vi "_Read.vi"(8 "error in (no error)":errorcluster, 11 "Lockin and Fluke Multimeter in":refnum<class "Lockin and Fluke Multimeter.lvclass">) -> (0 "error out":errorcluster, 2 "X array":T1, 3 "Lockin and Fluke Multimeter out":refnum<class "Lockin and Fluke Multimeter.lvclass">)   [LabVIEW 2017, in "Lockin and Fluke Multimeter.lvclass"]
doc: "(Protected, Dynamic, Pure Virtual/Abstract) Perform a measurement and return one or more channels of data. Outsiders should not call this method, but instead the public \"Read Data.vi\"."
uses:
  Lockin and Fluke Multimeter.lvclass
  Utility Classes/Readable/X array.ctl
  Utility Classes/Readable/X.ctl
  Lockin and Fluke Multimeter.lvclass/Lockin and Fluke Multimeter.ctl
  Lockin/sr830/SR830.lvlib
  Fluke Multimeter/Fluke 8840/Fluke 8840.lvlib
  Utility Classes/Readable/Readable.lvclass
panel:
  out "Ratio multiplier":dbl
  out "Fluke multiplier":dbl
  out "Lockin multiplier":dbl
  out "Fluke measurement":dbl format="%^.6e"
  out "R":dbl
  out "Y":dbl
  out "X":dbl
  out "trigger mode (0:internal)":u16(ring) items=["internal - continuous trigger", "external - rear panel trigger with delay", "external - bus trigger with delay", "external - rear panel trigger", "external - bus trigger"]
  out "rate (0:slow)":u16(ring) items=["slow", "medium", "fast"]
  out "range (0:auto)":u16(ring) items=["autorange", "200mV, 200 ohms", "2V, 2 kohms", "20V, 20 kohms", "200V, 200 kohms", "1000Vdc, 700 Vac, 2 Mohms", "20 Mohms"]
  out "function (0:volts DC)":u16(ring) items=["volts DC", "volts AC", "2-wire k.ohms", "4-wire k.ohms", "mA DC", "mA AC"]
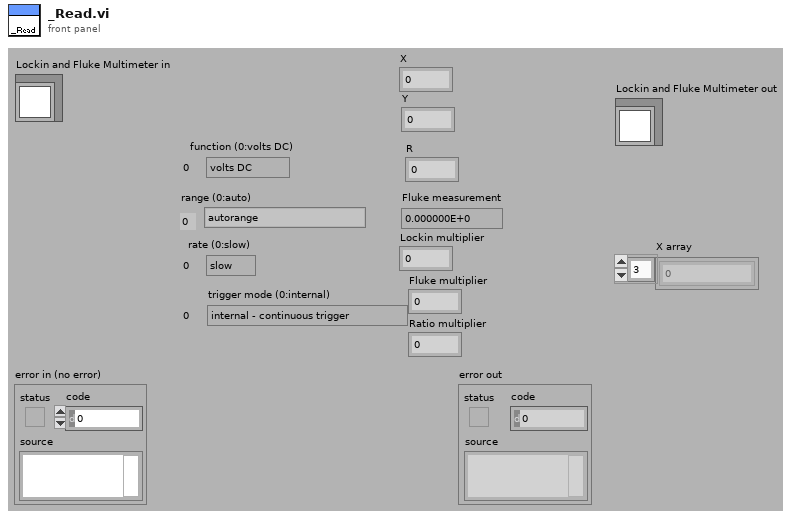
[diagram p1: front panel]
types:
  T1 = typedef "Readable.lvclass/X array.ctl" = T2[]
  T2 = typedef "Readable.lvclass/X.ctl" = dbl
  T3 = typedef "Lockin SR830.lvclass/Sensitivity.ctl" = u16
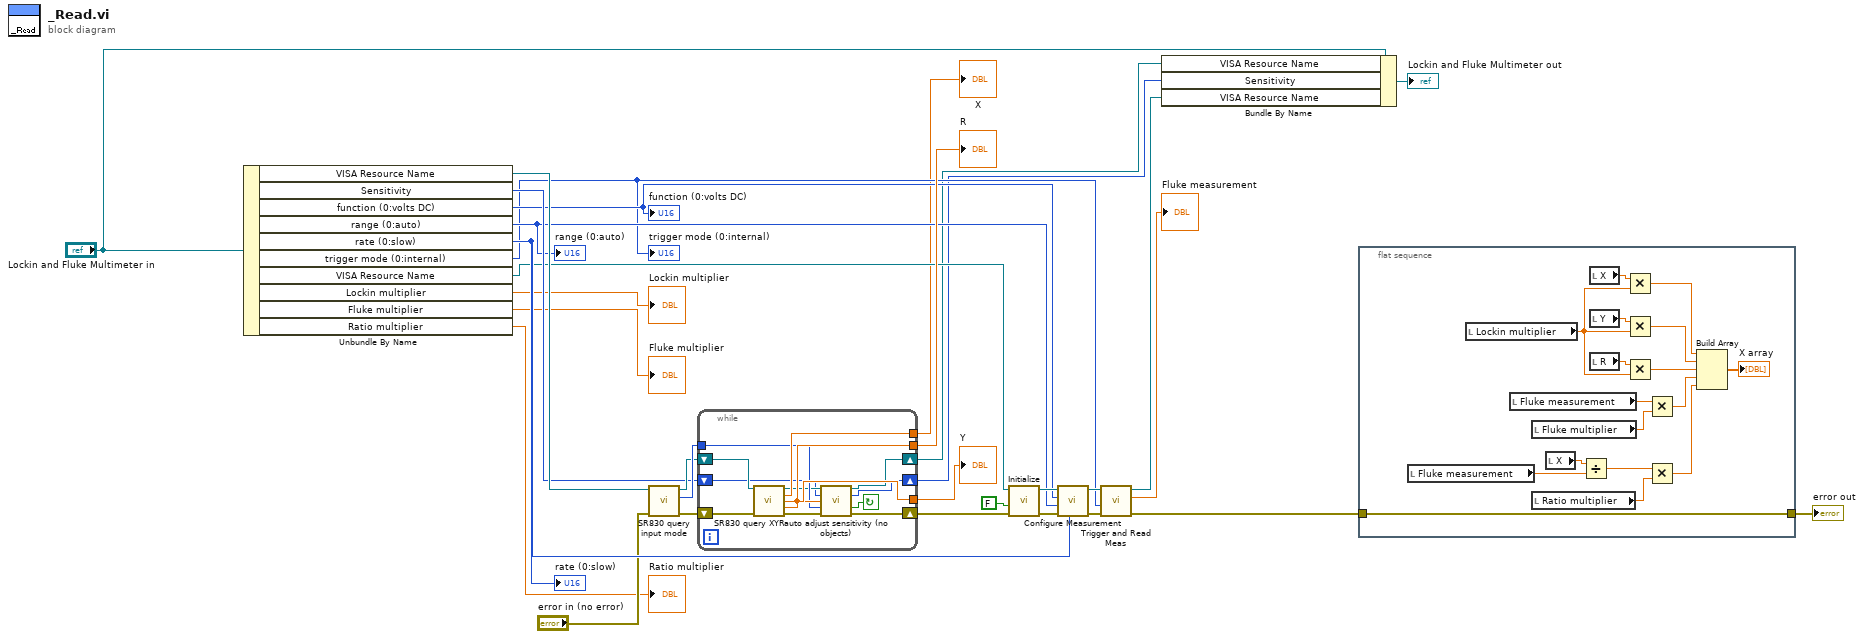
[diagram p0: block diagram]
diagram:
  n1 = Unbundle By Name("Lockin and Fluke Multimeter in") -> ("VISA Resource Name"=w28:refnum<visa-resource-name>, "Sensitivity"=w27:T3, "function (0:volts DC)"=w22:u16, "range (0:auto)"=w21:u16, "rate (0:slow)"=w20:u16, "trigger mode (0:internal)"=w19:u16, "VISA Resource Name"=w18:refnum<visa-resource-name>, "Lockin multiplier"=→"Lockin multiplier":dbl, "Fluke multiplier"=→"Fluke multiplier":dbl, "Ratio multiplier"=→"Ratio multiplier":dbl)
  "function (0:volts DC)" <- w22
  "range (0:auto)" <- w21
  "rate (0:slow)" <- w20
  "trigger mode (0:internal)" <- w19
  n2 = call "SR830 query input mode.vi"("error in (no error)"="error in (no error)", "VISA resource name"=w28) -> ("error out"=w29:errorcluster, "input mode"=w31:enum16{"A", "A-B", "I (10^6)", "I (10^8)"}, "VISA resource name out"=w30:refnum<visa-resource-name>)  [unwired: 7 in]
  n3 = while {
    tunnel: w31 -> [w39]
    shift-right: [w32] -> w15
    shift-left: w27 -> [w33]
    shift-right: [w36] -> w11
    shift-left: w29 -> [w44]
    shift-right: [w34] -> w16
    shift-left: w30 -> [w43]
    tunnel: [w42] -> w14
    tunnel: [w41] -> w26
    tunnel: [w40] -> w25
    stop <- w37 continue-if-true
    n4 = call "SR830 query XYR.vi"("VISA resource name"=w43, "error in (no error)"=w44) -> ("VISA resource name out"=w35:refnum<visa-resource-name>, "X"=w42:dbl, "Y"=w41:dbl, "R"=w40:dbl, "error out"=w38:errorcluster)  [unwired: 9 in]
    n5 = call "auto adjust sensitivity (no objects).vi"("VISA Resource Name"=w35, "sensitivity"=w33, "R value"=w40, "Input Setting"=w39, "error in (no error)"=w38) -> ("VISA resource name out"=w34:refnum<visa-resource-name>, "sensitivity out"=w32:i8, "Repeat Measurement?"=w37:bool, "error out"=w36:errorcluster)  [unwired: 7 in]
  }
  "X" <- w14
  "Y" <- w26
  "R" <- w25
  n6 = call "Initialize.vi"("error in (no error)"=w11, "reset (T:yes)"=FALSE, "VISA resource name"=w18) -> ("error out"=w10:errorcluster, "VISA resource name out"=w24:refnum<visa-resource-name>)  [unwired: 7 out]
  n7 = call "Configure Measurement.vi"("rate (0:slow)"=w20, "error in (no error)"=w10, "range (0:auto)"=w21, "function (0:volts DC)"=w22, "VISA resource name"=w24) -> ("error out"=w9:errorcluster, "VISA resource name out"=w23:refnum<visa-resource-name>)  [unwired: 5 out]
  n8 = call "Trigger and Read Meas.vi"("error in (no error)"=w9, "trigger mode (0:internal)"=w19, "VISA resource name"=w23) -> ("error out"=w1:errorcluster, "measurement"=→"Fluke measurement":dbl, "VISA resource name out"=w17:refnum<visa-resource-name>)  [unwired: 6 out]
  n9 = Bundle By Name(cluster="Lockin and Fluke Multimeter in", "VISA Resource Name"=w16, "Sensitivity"=w15, "VISA Resource Name"=w17) -> (→"Lockin and Fluke Multimeter out":refnum<class "Lockin and Fluke Multimeter.lvclass">)
  n10 = flat-sequence {
    tunnel: [w45] -> w2
    tunnel: w1 -> [w45]
    frame #0 {
      n11 = local read "Fluke measurement"() -> (w52:dbl)
      n12 = local read "Lockin multiplier"() -> (w57:dbl)
      n13 = local read "Fluke measurement"() -> (w47:dbl)
      n14 = local read "Fluke multiplier"() -> (w48:dbl)
      n15 = local read "Ratio multiplier"() -> (w50:dbl)
      n16 = local read "X"() -> (w53:dbl)
      n17 = Divide(x=w53, y=w52) -> (x/y=w51:dbl)
      n18 = local read "X"() -> (w60:dbl)
      n19 = local read "Y"() -> (w59:dbl)
      n20 = local read "R"() -> (w58:dbl)
      n21 = Multiply(x=w60, y=w57) -> (x*y=w56:dbl)
      n22 = Multiply(x=w59, y=w57) -> (x*y=w55:dbl)
      n23 = Multiply(x=w58, y=w57) -> (x*y=w54:dbl)
      n24 = Multiply(x=w47, y=w48) -> (x*y=w46:dbl)
      n25 = Multiply(x=w51, y=w50) -> (x*y=w49:dbl)
      n26 = Build Array(w56, w55, w54, w46, w49) -> (→"X array":dbl[])
    }
  }
  "error out" <- w2
